vi "Ardunio.vi"() -> ()   [LabVIEW 2017]
uses:
  C:/Users/mjoha/Documents/School/ELIC328/LabViewProject/builds/StatusVI/Server Status/mjohansen.labview.email.dll
  builds/StatusVI/Server Status/mjohansen.labview.email.dll
  <vilib>/MakerHub/LINX/Public/Peripherals/Digital/Digital Write 1 Chan.vi
  <vilib>/MakerHub/LINX/Public/Peripherals/Digital/Digital Write N Chans.vi
  <vilib>/MakerHub/LINX/Private/Local IO/LinxDigitalWrite.vi
  <vilib>/MakerHub/LINX/Public/Utilities/Check Channel.vi
  <vilib>/MakerHub/LINX/Public/Utilities/Open Serial.vi
  Global 1.vi
  Global 3.vi
  <vilib>/MakerHub/LINX/Public/Sensors/Temperature/TMP3x/TMP35.vi
  <vilib>/MakerHub/LINX/Private/Utilties/Generate Error.vi
  <vilib>/MakerHub/LINX/LMH-LINX.lvlib
  <vilib>/MakerHub/LINX/Public/Sensors/Temperature/TMP3x/TMP3x.lvlib
panel:
  in  "Update Interval":u32
  in  "Push Notifications":bool
  out "Waveform Chart":T1(graph)
  out "Error Out":errorcluster
  in  "Average High":dbl
  in  "Zone 4 High":dbl
  in  "Zone 3 High":dbl
  in  "Zone 2 High":dbl
  in  "Zone 1 High":dbl
  out "Alarm":bool
  in  "Average Low":dbl
  out "Avgerage Temp":dbl(slide) scale=0.0..100.0
  out "Zone 4 Temp":dbl(slide) scale=0.0..100.0
  out "Zone 3 Temp":dbl(slide) scale=0.0..100.0
  out "Zone 2 Temp":dbl(slide) scale=0.0..100.0
  out "Zone 1 Temp":dbl(slide) scale=0.0..100.0
  in  "Monitoring":bool
  in  "Zone 4 Low":dbl
  in  "Zone 3 Low":dbl
  in  "Zone 2 Low":dbl
  in  "Zone 1 Low":dbl
  in  "Serial Port":refnum<visa-resource-name>
  # "Settings"
  # "Thresholds"
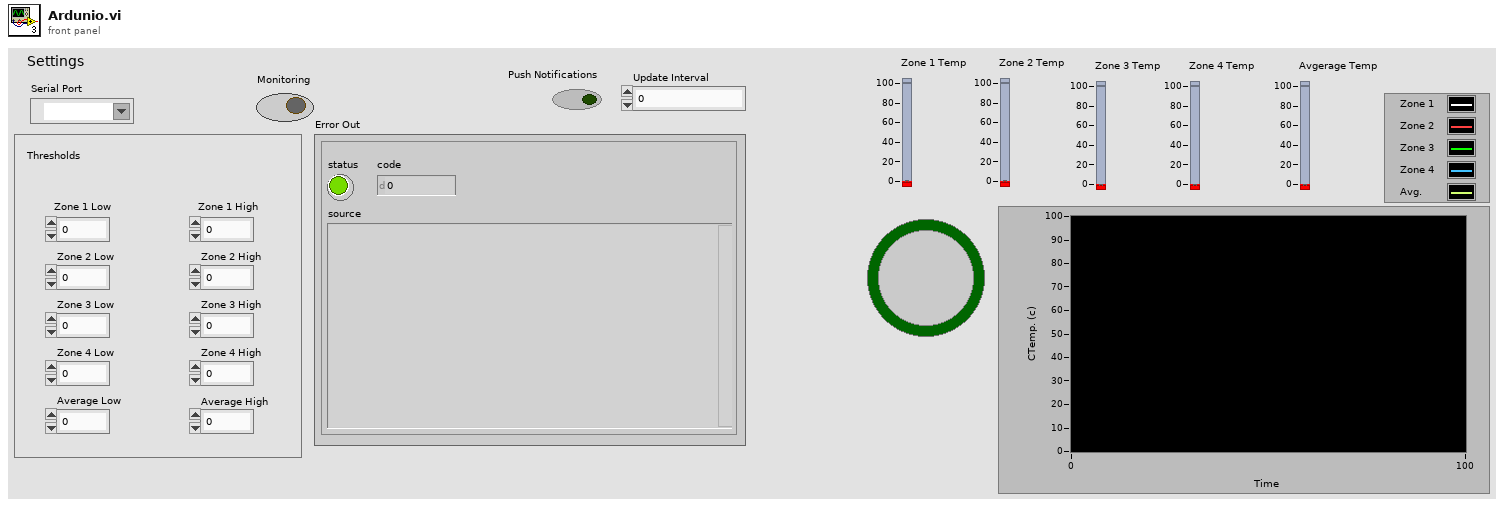
[diagram p1: front panel]
types:
  T1 = cluster{"Temp C":dbl, "Temp C":dbl, "Temp C":dbl, "Temp C":dbl, dbl}
  T2 = typedef "LMH-LINX.lvlib/LINX Ref.ctl" = cluster{"IO":T3, "Interface":T4, "LINX Device Config":T5}
  T3 = typedef "LMH-LINX.lvlib/Platform.ctl" = enum16{"Remote", "Local"}
  T4 = typedef "LMH-LINX.lvlib/Interface.ctl" = enum16{"Serial", "TCP"}
  T5 = typedef "LMH-LINX.lvlib/Device.lvlib/LINX Device Config.ctl" = cluster{"Interface":T4, "COM Port":refnum<visa-resource-name>, "TCP Configuration":T6, "Device Family":u8, "Device ID":u8, "Device Name":string, "TCP Ref":refnum<k5>, "Channels":T7}
  T6 = typedef "LMH-LINX.lvlib/Device.lvlib/TCP Config.ctl" = cluster{"IP Address":string, "Port":u16}
  T7 = typedef "LMH-LINX.lvlib/Channels.ctl" = cluster{"DI":u8[], "DO":u8[], "AI":u8[], "AO":u8[], "PWM":u8[], "QE":u8[], "UART":u8[], "I2C 2":u8[], "SPI":u8[], "CAN":u8[], "Servo":u8[], "AI Ref (V)":dbl, "AI Resolution (Bits)":u8, "AO Ref (V)":dbl, "AO Resolution (Bits)":u8}
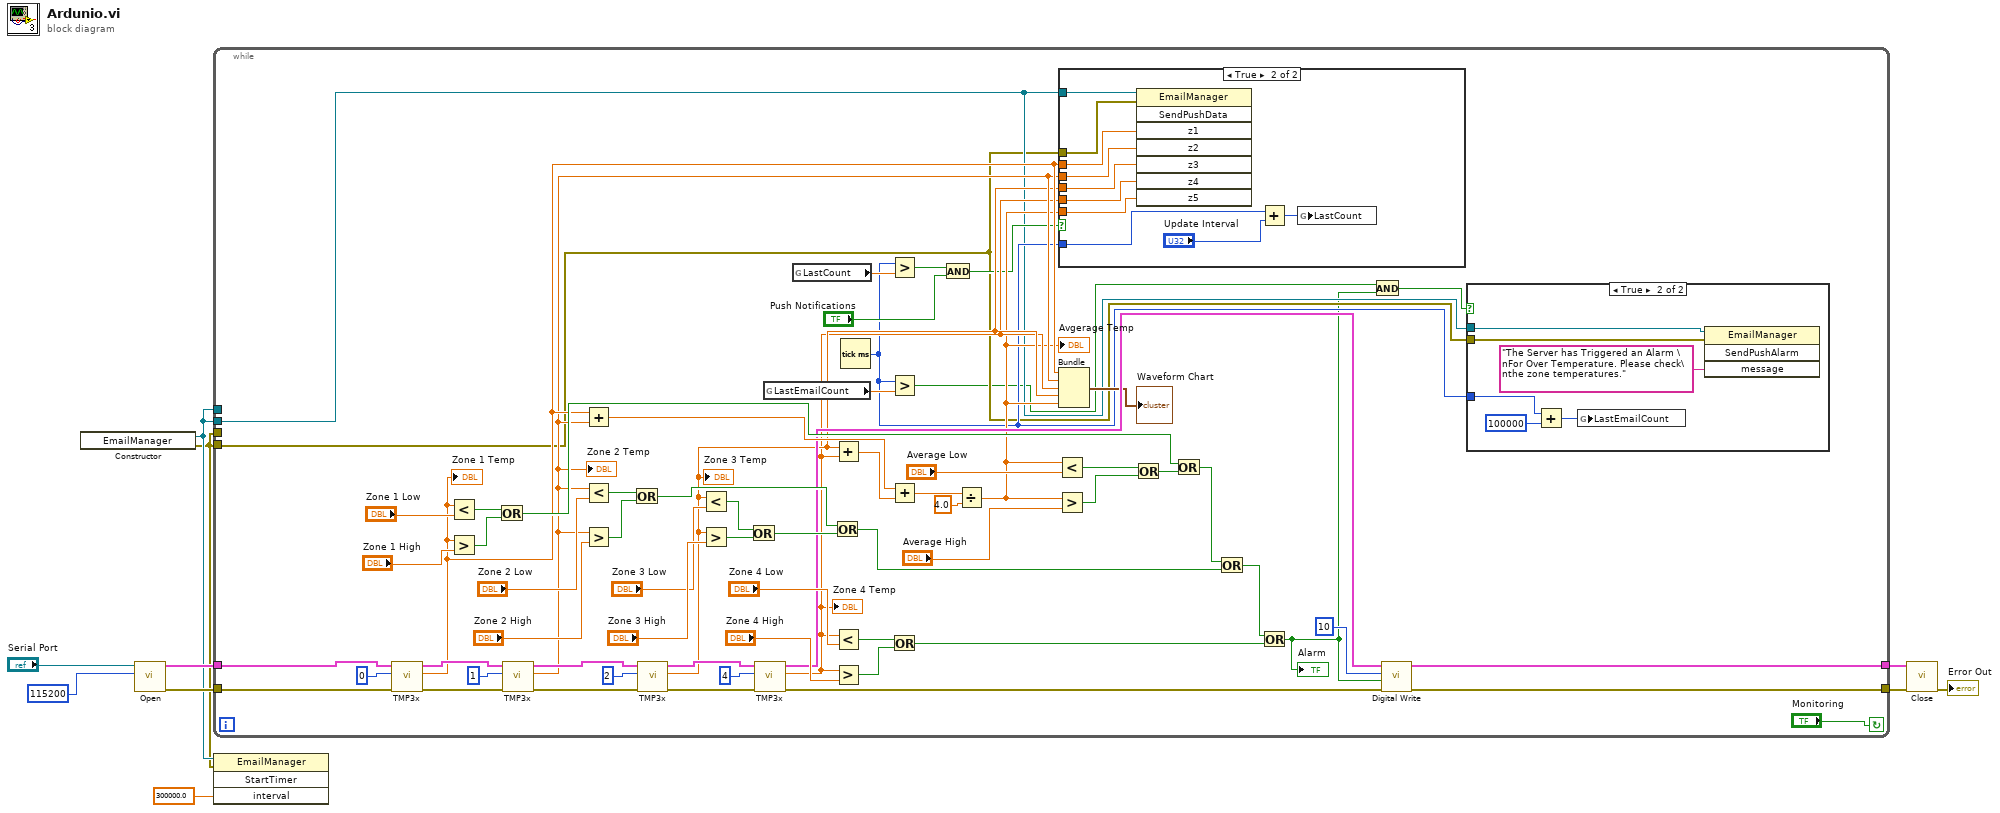
[diagram p0: block diagram]
diagram:
  n1 = constructor class="EmailManager"() -> (reference out=w2:refnum<k24>, error out=w1:errorcluster)  [unwired: 3 in, 1 out]
  n2 = call-poly <vilib>:"Open.vi"("Baud Rate Override"=u32 115200, "Serial Port"="Serial Port") -> ("Error Out"=w7:errorcluster, "LINX Resource"=w8:T2)  [unwired: 7 in, 1 out]
  n3 = while {
    tunnel: w8 -> [w72]
    tunnel: w7 -> [w76]
    tunnel: [w33] -> w6
    tunnel: [w32] -> w5
    tunnel: w2 -> [_]
    tunnel: w1 -> [_]
    tunnel: w2 -> [w15]
    tunnel: w1 -> [w14]
    stop <- "Monitoring" continue-if-true
    n4 = call-poly <vilib>:"TMP3x.vi"("Error In"=w76, "Analog Channel"=u8 0, "LINX Resource"=w72) -> ("Error Out"=w70:errorcluster, "Temp C"=w25:dbl, "LINX Resource"=w71:T2)  [unwired: 6 in]
    "Zone 1 Temp" <- w25
    n5 = Less?(x=w25, y="Zone 1 Low") -> (x < y?=w59:bool)
    n6 = Greater?(x=w25, y="Zone 1 High") -> (0:w58:bool)
    n7 = Or(x=w59, y=w58) -> (x .or. y?=w38:bool)
    n8 = call-poly <vilib>:"TMP3x.vi"("Error In"=w70, "Analog Channel"=u8 1, "LINX Resource"=w71) -> ("Error Out"=w68:errorcluster, "Temp C"=w24:dbl, "LINX Resource"=w69:T2)  [unwired: 6 in]
    "Zone 2 Temp" <- w24
    n9 = Add(x=w25, y=w24) -> (x+y=w65:dbl)
    n10 = Less?(x=w24, y="Zone 2 Low") -> (x < y?=w56:bool)
    n11 = Greater?(x=w24, y="Zone 2 High") -> (0:w55:bool)
    n12 = Or(x=w56, y=w55) -> (x .or. y?=w41:bool)
    n13 = call-poly <vilib>:"TMP3x.vi"("Error In"=w68, "Analog Channel"=u8 2, "LINX Resource"=w69) -> ("Error Out"=w66:errorcluster, "Temp C"=w23:dbl, "LINX Resource"=w67:T2)  [unwired: 6 in]
    "Zone 3 Temp" <- w23
    n14 = Less?(x=w23, y="Zone 3 Low") -> (x < y?=w53:bool)
    n15 = Greater?(x=w23, y="Zone 3 High") -> (0:w52:bool)
    n16 = Or(x=w53, y=w52) -> (x .or. y?=w40:bool)
    n17 = call-poly <vilib>:"TMP3x.vi"("Error In"=w66, "Analog Channel"=u8 4, "LINX Resource"=w67) -> ("Error Out"=w30:errorcluster, "Temp C"=w22:dbl, "LINX Resource"=w31:T2)  [unwired: 6 in]
    "Zone 4 Temp" <- w22
    n18 = global read "Global 3.vi" "LastEmailCount"() -> (w17:dbl)
    n19 = global read "Global 1.vi" "LastCount"() -> (w26:dbl)
    n20 = Or(x=w41, y=w40) -> (x .or. y?=w43:bool)
    n21 = Add(x=w23, y=w22) -> (x+y=w64:dbl)
    n22 = Less?(x=w22, y="Zone 4 Low") -> (x < y?=w51:bool)
    n23 = Greater?(x=w22, y="Zone 4 High") -> (0:w50:bool)
    n24 = Tick Count (ms)() -> (millisecond timer value=w16:u32)
    n25 = Greater?(x=w16, y=w26) -> (0:w20:bool)
    n26 = Greater?(x=w16, y=w17) -> (0:w13:bool)
    n27 = Add(x=w65, y=w64) -> (x+y=w63:dbl)
    n28 = Or(x=w51, y=w50) -> (x .or. y?=w39:bool)
    n29 = And(x=w20, y="Push Notifications") -> (x .and. y?=w18:bool)
    n30 = Divide(x=w63, y=4.0) -> (x/y=w21:dbl)
    "Avgerage Temp" <- w21
    n31 = Less?(x=w21, y="Average Low") -> (x < y?=w47:bool)
    n32 = Greater?(x=w21, y="Average High") -> (0:w46:bool)
    n33 = case shown="True" w18 {
      tunnel: w16 -> [_ w93]
      tunnel: w15 -> [_ w91]
      tunnel: w14 -> [_ w90]
      tunnel: w25 -> [_ w89]
      tunnel: w24 -> [_ w88]
      tunnel: w23 -> [_ w87]
      tunnel: w22 -> [_ w86]
      tunnel: w21 -> [_ w85]
      frame False {
      }
      frame True {
        n34 = invoke class="EmailManager" method="SendPushData"(reference=w91, error in=w90, "z1"=w89, "z2"=w88, "z3"=w87, "z4"=w86, "z5"=w85) -> ()  [unwired: 1 in, 8 out]
        n35 = Add(x=w93, y="Update Interval") -> (x+y=w92:u32)
        n36 = global write "Global 1.vi" "LastCount"(w92) -> ()
      }
    }
    n37 = Bundle("Temp C"=w25, "Temp C"=w24, "Temp C"=w22, "Temp C"=w23, w21) -> (→"Waveform Chart":T1)  [unwired: 1 in]
    n38 = Or(x=w47, y=w46) -> (x .or. y?=w45:bool)
    n39 = Or(x=w38, y=w45) -> (x .or. y?=w44:bool)
    n40 = Or(x=w44, y=w43) -> (x .or. y?=w42:bool)
    n41 = Or(x=w42, y=w39) -> (x .or. y?=w12:bool)
    "Alarm" <- w12
    n42 = And(x=w13, y=w12) -> (x .and. y?=w11:bool)
    n43 = call-poly <vilib>:"Digital Write.vi"("Error In"=w30, "Output Value"=w12, "DO Channel"=u8 10, "LINX Resource"=w31) -> ("Error Out"=w32:errorcluster, "LINX Resource"=w33:T2)  [unwired: 6 in]
    n44 = case shown="True" w11 {
      tunnel: w16 -> [_ w82]
      tunnel: w15 -> [_ w80]
      tunnel: w14 -> [_ w79]
      frame False {
      }
      frame True {
        n45 = Add(x=w82, y=u32 100000) -> (x+y=w83:u32)
        n46 = global write "Global 3.vi" "LastEmailCount"(w83) -> ()
        n47 = invoke class="EmailManager" method="SendPushAlarm"(reference=w80, error in=w79, "message"="The Server has Triggered an Alarm \nFor Over Temperature. Please check\nthe zone temperatures.") -> ()  [unwired: 1 in, 4 out]
      }
    }
  }
  n48 = invoke class="EmailManager" method="StartTimer"(reference=w2, error in=w1, "interval"=300000.0) -> ()  [unwired: 1 in, 4 out]
  n49 = call <vilib>:"Close.vi"("Error In"=w5, "LINX Resource"=w6) -> ("Error Out"=→"Error Out":errorcluster)  [unwired: 9 in]
